vi "Example.vi"() -> ()   [LabVIEW 2017]
uses:
  Child 2/Child 2.lvclass
  C:/LabVIEW Packages/Sources/Presentations/Inheritance/Parent/Parent.lvclass
  Child 1/Child 1.lvclass
  Parent/Parent.lvclass
panel:
  out "Array":string[](array[string])
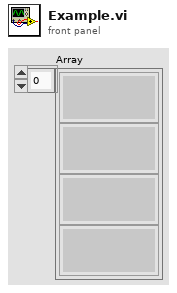
[diagram p1: front panel]
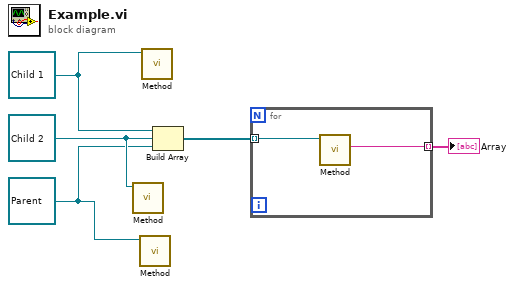
[diagram p0: block diagram]
diagram:
  w1 = refnum<class "Parent.lvclass"> refnum ("Parent.lvclass")
  w3 = refnum<class "Child 1.lvclass"> refnum ("Child 1.lvclass")
  w2 = refnum<class "Child 2.lvclass"> refnum ("Child 2.lvclass")
  n1 = call-dynamic "Method.vi"("Child 2 in"=w2) -> ()  [unwired: 8 in, 3 out]
  n2 = call-dynamic "Method.vi"("Parent in"=w1) -> ()  [unwired: 8 in, 3 out]
  n3 = call-dynamic "Method.vi"("Child 1 in"=w3) -> ()  [unwired: 8 in, 3 out]
  n4 = Build Array(w3, w2, w1) -> (w5:refnum<class "Parent.lvclass">[])
  n5 = for {
    tunnel: w5 -> [w7] mode=indexing
    tunnel: [w6] -> w4 mode=indexing
    n6 = call-dynamic "Method.vi"("Parent in"=w7) -> ("Output"=w6:string)  [unwired: 8 in, 2 out]
  }
  "Array" <- w4
